vi "myRIO_BRig_Host_endExp_getExp.vi"(11 "input_filePath":path) -> (2 "output_expPrefix":string)   [LabVIEW 2014]
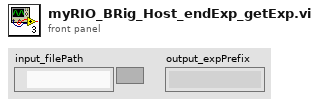
[diagram p1: front panel]
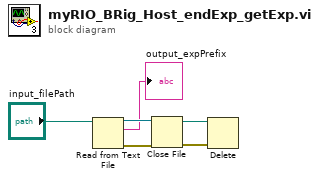
[diagram p0: block diagram]
diagram:
  n1 = Read from Text File(file (use dialog)="input_filePath") -> (refnum out=w6:refnum<file>, text=→"output_expPrefix":string, error out=w5:errorcluster)  [unwired: 3 in, 1 out]
  n2 = Close File(refnum=w6, error in=w5) -> (path=w2:path, error out=w1:errorcluster)
  n3 = Delete(path (use dialog)=w2, error in=w1) -> ()  [unwired: 3 in, 3 out]
